vi "DER Info Data from INI.vi"(8 "error in":errorcluster, 11 "Config Refnum in":T1) -> (0 "error out":errorcluster, 3 "Config Refnum out":T1, 4 "DER_Info":T2)   [LabVIEW 2018]
uses:
  <vilib>/ORNL/CSEISMIC DDS/CSEISMIC DDS Base/Data Types/DER_Info.ctl
  <vilib>/ORNL/CSEISMIC DDS/CSEISMIC DDS Base/Data Types/Controls/DeviceID.ctl
  <vilib>/Utility/config.llb/Config Data RefNum.ctl
  <vilib>/Utility/config.llb/Read Key (Double).vi
  <vilib>/Utility/config.llb/Read Key (String).vi
  <vilib>/Utility/config.llb/Read Key (U32).vi
  <vilib>/Utility/config.llb/Read Key (Boolean).vi
  <vilib>/ORNL/CSEISMIC DDS/CSEISMIC DDS Base/CSEISMIC DDS.lvclass
  <vilib>/Utility/config.llb/NI_LVConfig.lvlib
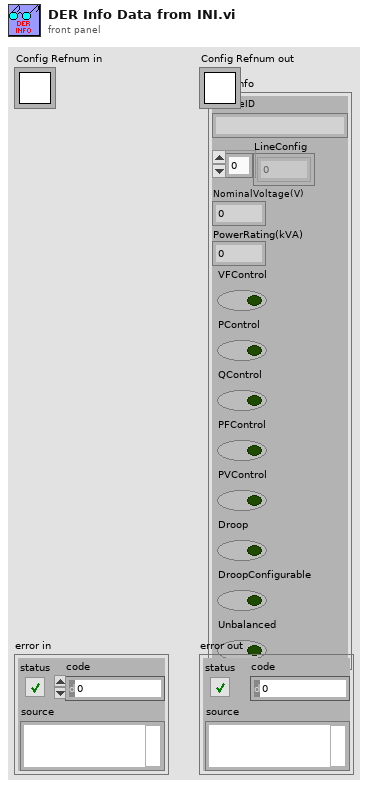
[diagram p1: front panel]
types:
  T1 = typedef "NI_LVConfig.lvlib/Config Data RefNum.ctl" = refnum<k1>
  T2 = typedef "CSEISMIC DDS.lvlib/CSEISMIC DDS.lvclass/DER_Info.ctl" = cluster{"DeviceID":T3, "LineConfig":u8[], "NominalVoltage(V)":dbl, "PowerRating(kVA)":dbl, "VFControl":bool, "PControl":bool, "QControl":bool, "PFControl":bool, "PVControl":bool, "Droop":bool, "DroopConfigurable":bool, "Unbalanced":bool}
  T3 = typedef "CSEISMIC DDS.lvlib/CSEISMIC DDS.lvclass/DeviceID.ctl" = string
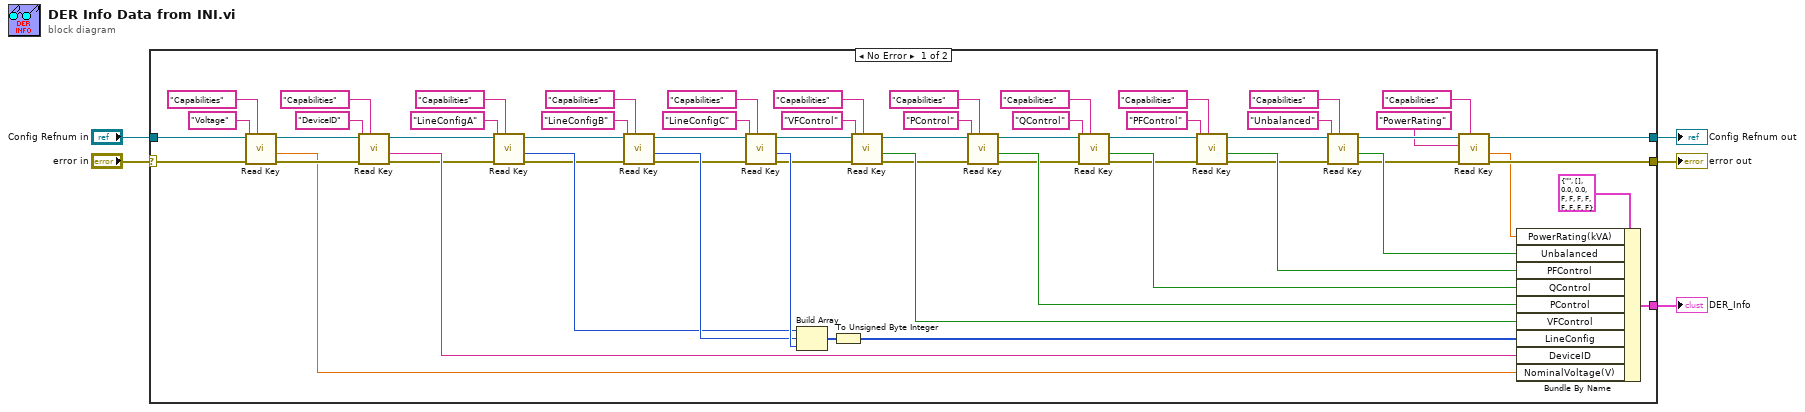
[diagram p0: block diagram]
diagram:
  n1 = case shown="No Error" "error in" {
    selector: "error in" -> [w14 w68]
    tunnel: [w66 _] -> w5
    tunnel: [w8 w68] -> w4
    tunnel: [w10 w67] -> w3
    tunnel: "Config Refnum in" -> [w17 w67]
    frame No Error {
      n2 = call-poly <vilib>:"Read Key.vi"("section"="Capabilities", "error in (no error)"=w14, "key"="Voltage", "refnum"=w17) -> ("error out"=w15:errorcluster, "value"=w13:dbl, "refnum out"=w16:T1)  [unwired: 4 in, 1 out]
      n3 = call-poly <vilib>:"Read Key.vi"("section"="Capabilities", "error in (no error)"=w15, "key"="DeviceID", "refnum"=w16) -> ("error out"=w57:errorcluster, "value"=w58:string, "refnum out"=w56:T1)  [unwired: 4 in, 1 out]
      n4 = call-poly <vilib>:"Read Key.vi"("section"="Capabilities", "error in (no error)"=w57, "key"="LineConfigA", "refnum"=w56) -> ("error out"=w45:errorcluster, "value"=w50:u32, "refnum out"=w44:T1)  [unwired: 4 in, 1 out]
      n5 = call-poly <vilib>:"Read Key.vi"("section"="Capabilities", "error in (no error)"=w45, "key"="LineConfigB", "refnum"=w44) -> ("error out"=w47:errorcluster, "value"=w51:u32, "refnum out"=w46:T1)  [unwired: 4 in, 1 out]
      n6 = call-poly <vilib>:"Read Key.vi"("section"="Capabilities", "error in (no error)"=w47, "key"="LineConfigC", "refnum"=w46) -> ("error out"=w49:errorcluster, "value"=w52:u32, "refnum out"=w48:T1)  [unwired: 4 in, 1 out]
      n7 = Build Array(w50, w51, w52) -> (w59:u32[])
      n8 = To Unsigned Byte Integer(number=w59) -> (unsigned 8bit integer=w60:u8[])
      n9 = call-poly <vilib>:"Read Key.vi"("section"="Capabilities", "error in (no error)"=w49, "key"="VFControl", "refnum"=w48) -> ("error out"=w36:errorcluster, "value"=w61:bool, "refnum out"=w32:T1)  [unwired: 4 in, 1 out]
      n10 = call-poly <vilib>:"Read Key.vi"("section"="Capabilities", "error in (no error)"=w36, "key"="PControl", "refnum"=w32) -> ("error out"=w37:errorcluster, "value"=w62:bool, "refnum out"=w33:T1)  [unwired: 4 in, 1 out]
      n11 = call-poly <vilib>:"Read Key.vi"("section"="Capabilities", "error in (no error)"=w37, "key"="QControl", "refnum"=w33) -> ("error out"=w38:errorcluster, "value"=w63:bool, "refnum out"=w34:T1)  [unwired: 4 in, 1 out]
      n12 = call-poly <vilib>:"Read Key.vi"("section"="Capabilities", "error in (no error)"=w38, "key"="PFControl", "refnum"=w34) -> ("error out"=w39:errorcluster, "value"=w64:bool, "refnum out"=w35:T1)  [unwired: 4 in, 1 out]
      n13 = call-poly <vilib>:"Read Key.vi"("section"="Capabilities", "error in (no error)"=w39, "key"="Unbalanced", "refnum"=w35) -> ("error out"=w9:errorcluster, "value"=w65:bool, "refnum out"=w11:T1)  [unwired: 4 in, 1 out]
      n14 = call-poly <vilib>:"Read Key.vi"("section"="Capabilities", "error in (no error)"=w9, "key"="PowerRating", "refnum"=w11) -> ("error out"=w8:errorcluster, "value"=w6:dbl, "refnum out"=w10:T1)  [unwired: 4 in, 1 out]
      n15 = Bundle By Name(cluster=T2 {"DeviceID"="", "LineConfig"=[], "NominalVoltage(V)"=0.0, "PowerRating(kVA)"=0.0, "VFControl"=FALSE, "PControl"=FALSE, "QControl"=FALSE, "PFControl"=FALSE, "PVControl"=FALSE, "Droop"=FALSE, "DroopConfigurable"=FALSE, "Unbalanced"=FALSE} ("DER_Info"), "PowerRating(kVA)"=w6, "Unbalanced"=w65, "PFControl"=w64, "QControl"=w63, "PControl"=w62, "VFControl"=w61, "LineConfig"=w60, "DeviceID"=w58, "NominalVoltage(V)"=w13) -> (w66:T2)
    }
    frame Error {
    }
  }
  "DER_Info" <- w5
  "error out" <- w4
  "Config Refnum out" <- w3
